vi "Get Interface.vi"(8 "error in (no error)":errorcluster, 11 "Output Actor Hardware in":refnum<class "Output Actor Hardware.lvclass">) -> (0 "error out":errorcluster, 2 "Output Actor Interface":refnum<class "Output Actor Interface.lvclass">, 3 "Output Actor Hardware out":refnum<class "Output Actor Hardware.lvclass">)   [LabVIEW 2015, in "Output Actor Hardware.lvclass"]
uses:
  Output Actor Hardware.lvclass
  Output Actor/Output Actor Interface/Output Actor Interface.lvclass
  Output Actor Hardware Interface/Output Actor Hardware Interface.lvclass
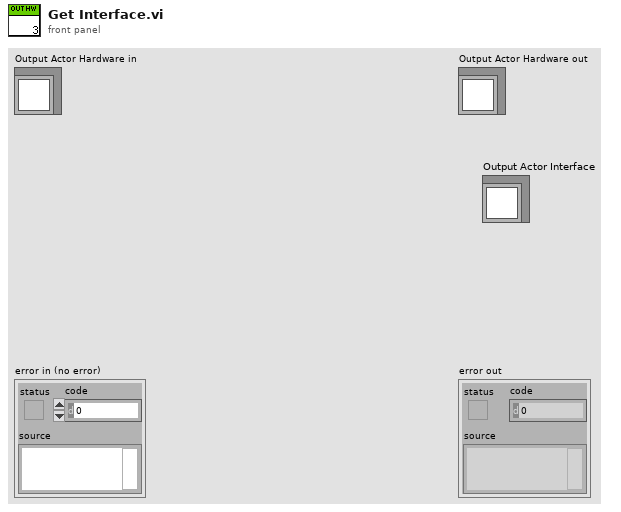
[diagram p1: front panel]
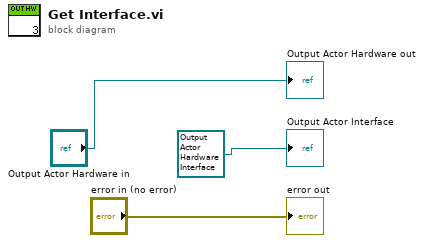
[diagram p0: block diagram]
diagram:
  "error out" <- "error in (no error)"
  "Output Actor Hardware out" <- "Output Actor Hardware in"
  "Output Actor Interface" <- refnum<class "Output Actor Hardware Interface.lvclass"> refnum ("Output Actor Hardware Interface.lvclass")
